vi "Get Channel Names.vi"(8 "error in (no error)":errorcluster, 11 "IntanElectrophysiology in":refnum<class "IntanElectrophysiology.lvclass">) -> (0 "error out":errorcluster, 2 "Strings and Numbers":cluster{refnum<k21>, i32}[](array[cluster]), 3 "IntanElectrophysiology out":refnum<class "IntanElectrophysiology.lvclass">)   [LabVIEW 2014, in "IntanElectrophysiology.lvclass"]
uses:
  IntanElectrophysiology.lvclass
  IntanElectrophysiology.lvclass/IntanElectrophysiology.ctl
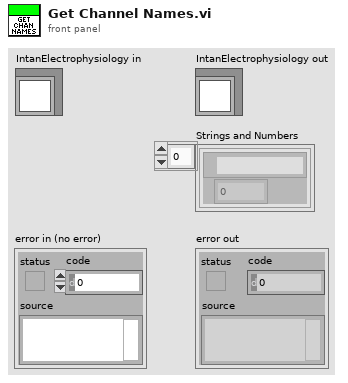
[diagram p1: front panel]
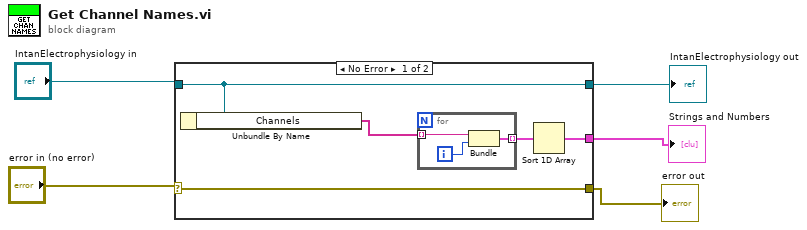
[diagram p0: block diagram]
diagram:
  n1 = case shown="No Error" "error in (no error)" {
    selector: "error in (no error)" -> [w8 w15]
    tunnel: [w8 w15] -> w3
    tunnel: [w7 w14] -> w5
    tunnel: "IntanElectrophysiology in" -> [w7 w14]
    tunnel: [w9 _] -> w4
    frame No Error {
      n2 = Unbundle By Name(w7) -> ("Channels"=w6:string[])
      n3 = for {
        tunnel: w6 -> [w13] mode=indexing
        tunnel: [w12] -> w10 mode=indexing
        i -> [w11]
        n4 = Bundle("Name"=w13, w11) -> (w12:cluster{"Name":string, i32})  [unwired: 1 in]
      }
      n5 = Sort 1D Array(array=w10) -> (sorted array=w9:cluster{"Name":string, i32}[])
    }
    frame Error {
    }
  }
  "error out" <- w3
  "IntanElectrophysiology out" <- w5
  "Strings and Numbers" <- w4
